vi "19_ВПТемпературныйМонитор.vi"() -> ()   [LabVIEW 2016]
panel:
  in  "Boolean":bool
  out "Waveform Chart":dbl(graph)
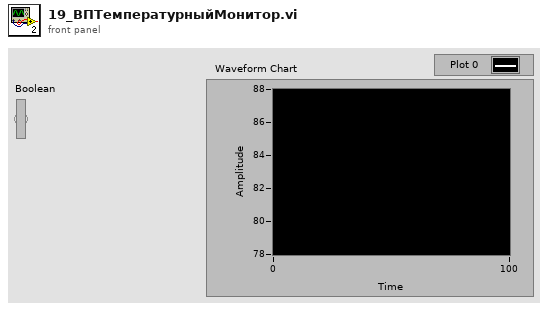
[diagram p1: front panel]
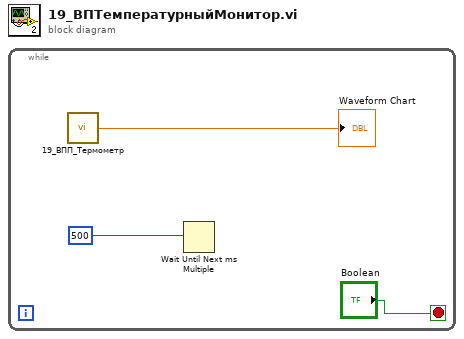
[diagram p0: block diagram]
diagram:
  n1 = while {
    stop <- "Boolean" stop-if-true
    n2 = call "19_ВПП_Термометр.vi"() -> ("Thermometer"=→"Waveform Chart":dbl)
    n3 = Wait Until Next ms Multiple(millisecond multiple=500) -> ()  [unwired: 1 out]
  }
